vi "LogaddSkipped.vi"(8 "error in (no error)":errorcluster, 11 "String in":refnum<vi>) -> (0 "error out":errorcluster)   [LabVIEW 2017]
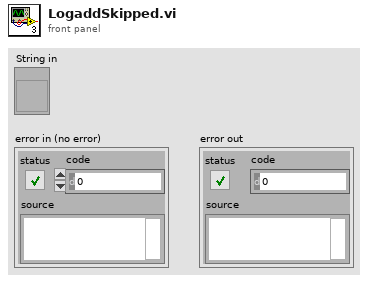
[diagram p1: front panel]
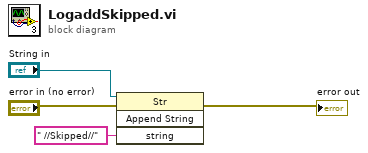
[diagram p0: block diagram]
diagram:
  n1 = invoke class="Str" method="Append String"(reference="String in", error in="error in (no error)", "string"=" //Skipped//") -> (error out=→"error out":errorcluster)  [unwired: 1 in, 3 out]
